vi "Read Shaft Length.vi"(11 "Prybar in":refnum<class "Prybar.lvclass">) -> (2 "length cm":dbl=100.0, 3 "Prybar out":refnum<class "Prybar.lvclass">)   [LabVIEW 2023, in "Prybar.lvclass"]
uses:
  Prybar.lvclass
  Prybar.lvclass/Prybar.ctl
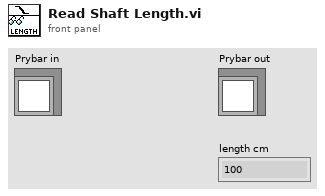
[diagram p1: front panel]
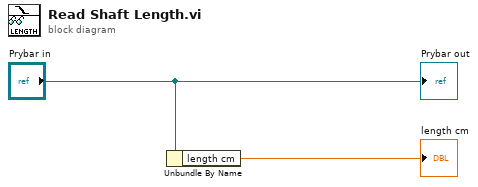
[diagram p0: block diagram]
diagram:
  n1 = Unbundle By Name("Prybar in") -> ("length cm"=→"length cm":dbl)
  "Prybar out" <- "Prybar in"
